vi "Write Manejador de turnos.vi"(8 "error in (no error)":errorcluster, 10 "Manejador de turnos":refnum<vi>, 11 "Manejo Turnos in":refnum<class "Manejo Turnos.lvclass">) -> (0 "error out":errorcluster, 3 "Manejo Turnos out":refnum<class "Manejo Turnos.lvclass">)   [LabVIEW 2020, in "Manejo Turnos.lvlib" / "Manejo Turnos.lvclass"]
uses:
  Manejo Turnos.lvclass
  Manejo Turnos.lvclass/Manejo Turnos.ctl
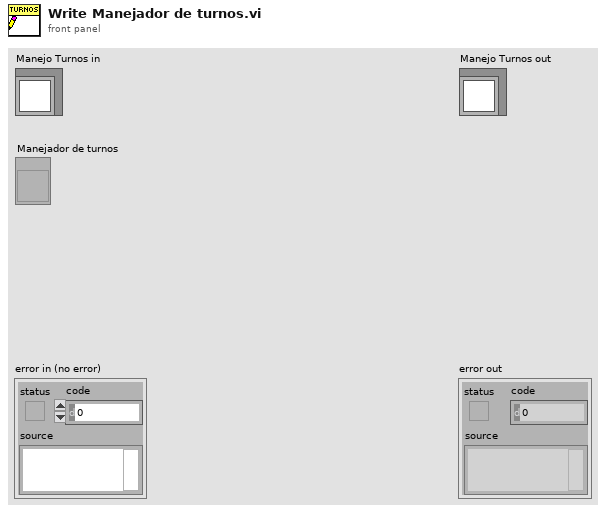
[diagram p1: front panel]
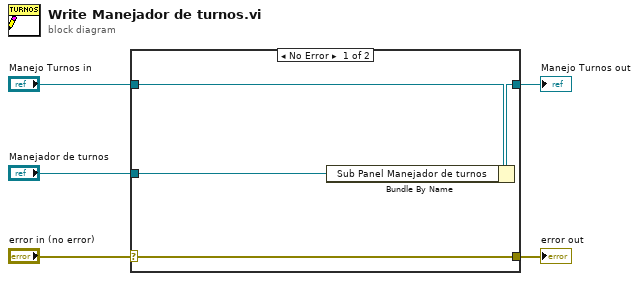
[diagram p0: block diagram]
diagram:
  n1 = case shown="No Error" "error in (no error)" {
    selector: "error in (no error)" -> [w9 w10]
    tunnel: [w9 w10] -> w4
    tunnel: [w7 w11] -> w2
    tunnel: "Manejo Turnos in" -> [w8 w11]
    tunnel: "Manejador de turnos" -> [w6 _]
    frame No Error {
      n2 = Bundle By Name(cluster=w8, "Sub Panel Manejador de turnos"=w6) -> (w7:refnum<class "Manejo Turnos.lvclass">)
    }
    frame Error {
    }
  }
  "error out" <- w4
  "Manejo Turnos out" <- w2
